vi "L0_MajnAdds_File_Appender.vi"(0 "Vin":dbl, 1 "CH":dbl, 2 "Att":dbl, 3 "IbClip":dbl=63.0, 4 "Clip":dbl=1.0, 5 "Vmeas":dbl, 7 "file path (dialog if empty)":path) -> ()   [LabVIEW 2009]
uses:
  <vilib>/Utility/file.llb/Write To Spreadsheet File (string).vi
panel:
  in  "Threshold":dbl=1.0
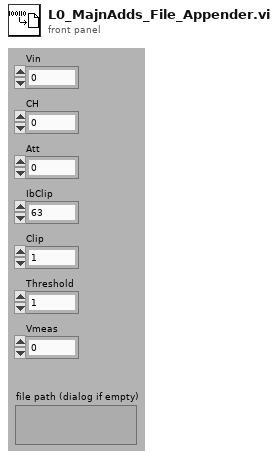
[diagram p1: front panel]
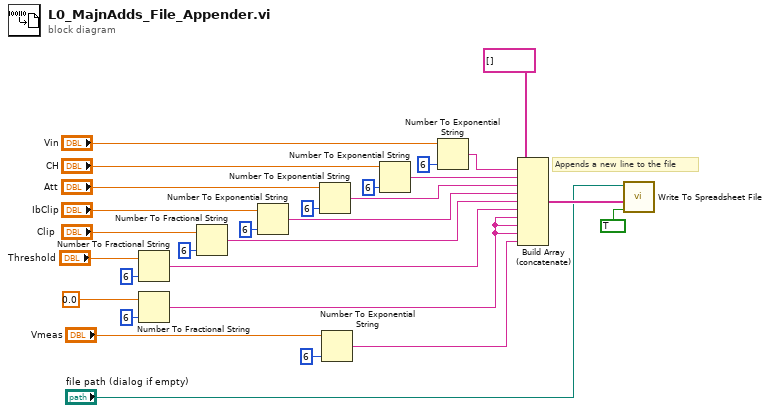
[diagram p0: block diagram]
diagram:
  # "Appends a new line to the file"
  n1 = Number To Fractional String(number="Threshold", precision (6)=i16 6) -> (F-format string=w1:string)  [unwired: 2 in]
  n2 = Number To Fractional String(number=0.0, precision (6)=i16 6) -> (F-format string=w4:string)  [unwired: 2 in]
  n3 = Number To Fractional String(number="Clip", precision (6)=i16 6) -> (F-format string=w21:string)  [unwired: 2 in]
  n4 = Number To Exponential String(number="IbClip", precision (6)=i16 6) -> (E-format string=w25:string)  [unwired: 2 in]
  n5 = Number To Exponential String(number="Att", precision (6)=i16 6) -> (E-format string=w27:string)  [unwired: 2 in]
  n6 = Number To Exponential String(number="Vmeas", precision (6)=i16 6) -> (E-format string=w13:string)  [unwired: 2 in]
  n7 = Number To Exponential String(number="CH", precision (6)=i16 6) -> (E-format string=w28:string)  [unwired: 2 in]
  n8 = Number To Exponential String(number="Vin", precision (6)=i16 6) -> (E-format string=w20:string)  [unwired: 2 in]
  n9 = Build Array (concatenate)(string[] [] ("array"), w20, w28, w27, w25, w21, w1, w4, w4, w4, w13) -> (w16:string[])
  n10 = call-poly <vilib>:"Write To Spreadsheet File.vi"("append to file? (new file:F)"=TRUE, "1D data"=w16, "file path (dialog if empty)"="file path (dialog if empty)") -> ()  [unwired: 5 in, 1 out]
